vi "Dequeue Message.vi"(8 "error in (no error)":errorcluster, 9 "timeout in ms (-1)":i32, 11 "Queue in":refnum<queue>) -> (0 "error out":errorcluster, 1 "Cmd":string, 2 "Data":variant, 3 "Queue out":refnum<queue>)   [LabVIEW 2016]
uses:
  Controls/Message Structure.ctl
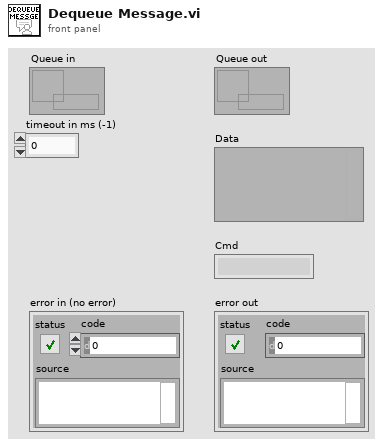
[diagram p1: front panel]
types:
  T1 = typedef "Message Structure.ctl" = cluster{"Data":variant, "Cmd":string}
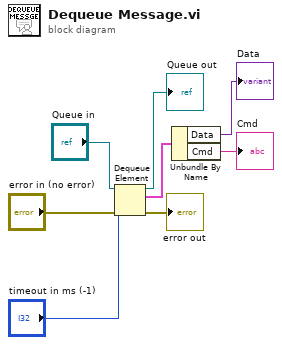
[diagram p0: block diagram]
diagram:
  n1 = Dequeue Element(queue="Queue in", timeout in ms (-1)="timeout in ms (-1)", error in (no error)="error in (no error)") -> (queue out=→"Queue out":refnum<queue>, element=w6:T1, error out=→"error out":errorcluster)  [unwired: 1 out]
  n2 = Unbundle By Name(w6) -> ("Data"=→"Data":variant, "Cmd"=→"Cmd":string)
